vi "LV_InflateStr.vi"(8 "error in (no error)":errorcluster, 11 "Deflated string with size header":string) -> (0 "error out":errorcluster, 3 "Inflated string":string)   [LabVIEW 2020]
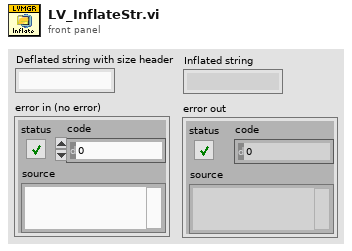
[diagram p1: front panel]
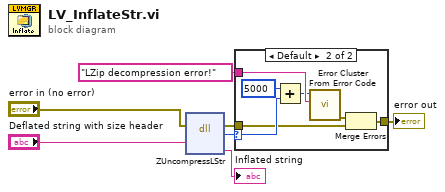
[diagram p0: block diagram]
diagram:
  n1 = dll-call lib="LabVIEW" fn="ZUncompressLStr"(error in="error in (no error)", "DeflatedString"="Deflated string with size header") -> (error out=w2:errorcluster, "return type"=w3:i32, "InflatedString"=→"Inflated string":string)  [unwired: 4 in, 1 out]
  n2 = case shown="Default" w3 {
    selector: w3 -> [_ w13]
    tunnel: "LZip decompression error!" ("error message (\"\")") -> [_ w15]
    tunnel: w2 -> [w8 w10]
    tunnel: [w8 w9] -> w1
    frame 0 {
    }
    frame Default {
      n3 = Add(x=5000, y=w13) -> (x+y=w14:i32)
      n4 = call <vilib>:"Error Cluster From Error Code.vi"("error message (\"\")"=w15, "error code (0)"=w14) -> ("error out"=w11:errorcluster)  [unwired: 7 in]
      n5 = Merge Errors(w11, w10) -> (w9:errorcluster)
    }
  }
  "error out" <- w1
